vi "Init Hardware.vi"(8 "error in (no error)":errorcluster, 11 "Red Pitaya Transceiver Driver in":refnum<class "Red Pitaya Transceiver Driver.lvclass">) -> (0 "error out":errorcluster, 3 "Red Pitaya Transceiver Driver out":refnum<class "Red Pitaya Transceiver Driver.lvclass">)   [LabVIEW 2016, in "Red Pitaya Transceiver Driver.lvclass"]
uses:
  Red Pitaya Transceiver Driver.lvclass
  RP Transceiver/Receiver format.ctl
  Red Pitaya Transceiver Driver.lvclass/Red Pitaya Transceiver Driver.ctl
  RP Instrument/RP Instrument.lvclass/RP Instrument.ctl
  RP Transceiver/RP Transceiver.lvclass/RP Transceiver.ctl
  Read RP Transceiver.vi
  RP Instrument/Write DDS delay.vi
  RP Transceiver/Write Receiver format.vi
  Write RP Transceiver.vi
  RP Transceiver/RP Transceiver.lvclass
  C:/github/NHMFL_Core/Libraries/Red Pitaya/RP Core/RP Instrument/RP Instrument.lvclass
  Read Spectrum Configuration.vi
  RP Instrument/Write Server address.vi
  Instruments/Instrument Driver/Instrument Driver.lvclass
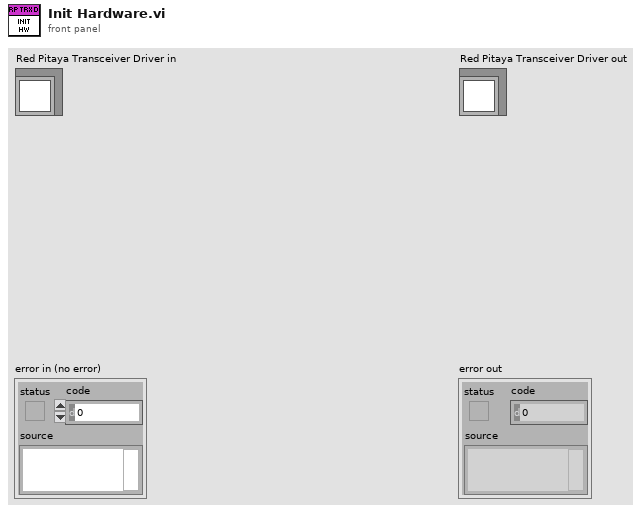
[diagram p1: front panel]
types:
  T1 = typedef "Receiver format.ctl" = enum16{"X-Y-F", "F-X-Y", "X-Y", "X"}
  T2 = typedef "Spectrum Configuration.ctl" = cluster{"Start frequency":dbl, "End frequency":dbl, "Coarse step":dbl, "Step duration":dbl, "Red Pitaya address":string, "Open plot \non start":bool, "Fine region centers":dbl[], "Regions width":dbl, "Fine step":dbl, "Pause between scans":dbl}
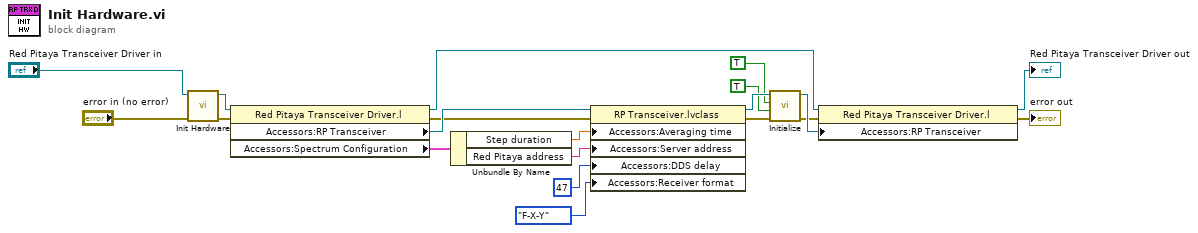
[diagram p0: block diagram]
diagram:
  n1 = call-parent "Init Hardware.vi"("error in (no error)"="error in (no error)", "Instrument Driver in"="Red Pitaya Transceiver Driver in") -> ("error out"=w20:errorcluster, "Instrument Driver out"=w17:refnum<class "Red Pitaya Transceiver Driver.lvclass">)  [unwired: 8 in]
  n2 = property class="Red Pitaya Transceiver Driver.l"(reference=w17, error in=w20) -> (reference out=w8:refnum<class "Red Pitaya Transceiver Driver.lvclass">, error out=w14:errorcluster, "Accessors:RP Transceiver"=w16:refnum<class "RP Transceiver.lvclass">, "Accessors:Spectrum Configuration"=w15:T2)
  n3 = Unbundle By Name(w15) -> ("Step duration"=w4:dbl, "Red Pitaya address"=w3:string)
  n4 = property class="RP Transceiver.lvclass"(reference=w16, error in=w14, "Accessors:Averaging time"=w4, "Accessors:Server address"=w3, "Accessors:DDS delay"=u32 47 ("DDS delay"), "Accessors:Receiver format"=Receiver_format."F-X-Y" ("Receiver format")) -> (reference out=w13:refnum<class "RP Transceiver.lvclass">, error out=w10:errorcluster)
  n5 = call-dynamic "Initialize.vi"("error in (no error)"=w10, "Send \"Connect client\""=TRUE ("Send \"Connect client\""), "Reset"=TRUE, "RP Transceiver in"=w13) -> ("error out"=w6:errorcluster, "RP Transceiver out"=w9:refnum<class "RP Transceiver.lvclass">)  [unwired: 6 in]
  n6 = property class="Red Pitaya Transceiver Driver.l"(reference=w8, error in=w6, "Accessors:RP Transceiver"=w9) -> (reference out=→"Red Pitaya Transceiver Driver out":refnum<class "Red Pitaya Transceiver Driver.lvclass">, error out=→"error out":errorcluster)
